vi "Get Multi.vi"(0 "Display State In":T2, 5 "Value In":T1, 9 "Container State":T3, 11 "error in (no error)":errorcluster) -> (4 "Display State Out":T2, 6 "Value Out":T1, 15 "error out":errorcluster)   [LabVIEW 2015, in "Vowel.xctl"]
uses:
  Vowel.xctl
  <vilib>/_xctls/Container State.ctl
  State.ctl
  Vowel.Properties.ctl
  Utility VIs/Controls/KCheckbox/KCheckbox.xctl
  <vilib>/_xctls/XControlSupport.lvlib
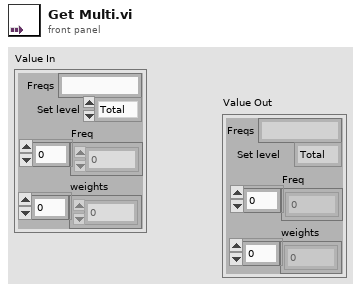
[diagram p1: front panel]
types:
  T1 = typedef "Vowel.xctl/Vowel.Properties.ctl" = cluster{"Freqs":string, "Set level":enum16{"Total", "Per component"}, "Freq":dbl[], "weights":dbl[]}
  T2 = typedef "Vowel.xctl/State.ctl" = cluster{"enable menu":bool, "ctls":cluster{"Freq":refnum<vi>, "Phase":refnum<vi>}}
  T3 = typedef "XControlSupport.lvlib/Container State.ctl" = cluster{"Indicator?":bool, "Run Mode?":bool, " Refnum":refnum<vi>}
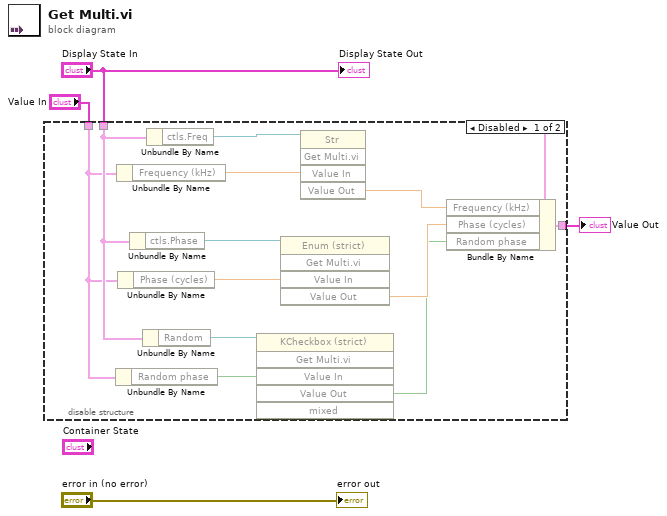
[diagram p0: block diagram]
diagram:
  n1 = disable-structure shown="Disabled" {
    disable-tunnel: [w16 w17] -> w3
    disable-tunnel: "Display State In" -> [w9 _]
    disable-tunnel: "Value In" -> [w8 w17]
    frame Disabled {
      n2 = Unbundle By Name(w8) -> ("Random phase"=w6:bool)
      n3 = Unbundle By Name(w8) -> ("Frequency (kHz)"=w13:dbl)
      n4 = Unbundle By Name(w8) -> ("Phase (cycles)"=w11:dbl)
      n5 = Unbundle By Name(w9) -> ("ctls.Phase"=w15:refnum<vi>)
      n6 = Unbundle By Name(w9) -> ("Random"=w7:refnum<vi>)
      n7 = Unbundle By Name(w9) -> ("ctls.Freq"=w14:refnum<vi>)
      n8 = invoke class="KCheckbox (strict)" method="Get Multi.vi"(reference=w7, "Value In"=w6) -> ("Value Out"=w5:bool)  [unwired: 4 in, 5 out]
      n9 = invoke class="Enum (strict)" method="Get Multi.vi"(reference=w15, "Value In"=w11) -> ("Value Out"=w10:dbl)  [unwired: 3 in, 4 out]
      n10 = invoke class="Str" method="Get Multi.vi"(reference=w14, "Value In"=w13) -> ("Value Out"=w12:dbl)  [unwired: 3 in, 4 out]
      n11 = Bundle By Name(cluster=w8, "Frequency (kHz)"=w12, "Phase (cycles)"=w10, "Random phase"=w5) -> (w16:T1)
    }
    frame Enabled {
    }
  }
  "Value Out" <- w3
  "Display State Out" <- "Display State In"
  "error out" <- "error in (no error)"
